vi "ReadRecords.vi"(8 "error in (no error)":errorcluster, 10 "Num records to read":i32, 11 "FpgaRef5782 in":refnum<class "FpgaRefx410.lvclass">) -> (0 "error out":errorcluster, 2 "Data":dbl[][](array[numeric]), 3 "FpgaRef5782 out":refnum<class "FpgaRefx410.lvclass">)   [LabVIEW 2025, in "FpgaRefx410.lvclass"]
uses:
  FpgaRefx410.lvclass
  FpgaRefx410.lvclass/FpgaRefx410.ctl
  <vilib>/Utility/error.llb/Error Cluster From Error Code.vi
  <vilib>/rvi/errors/niLvFpgaAdjustHostInterfaceError.vi
  <vilib>/rvi/interface/nirviMethod/nirviMethod.xnode
  x410 FPGA ref.ctl
  <vilib>/FPGAPlugInAG/Dynamic/niLvFpga_ReadFifo_Dynamic.vi
  <vilib>/rvi/errors/niLvFpgaMergeErrorWithErrorCode.vi
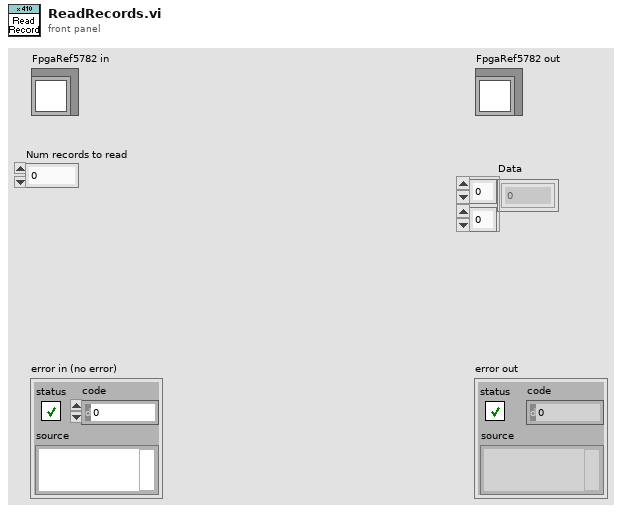
[diagram p1: front panel]
types:
  T1 = typedef "x410 FPGA ref.ctl" = refnum<k20>
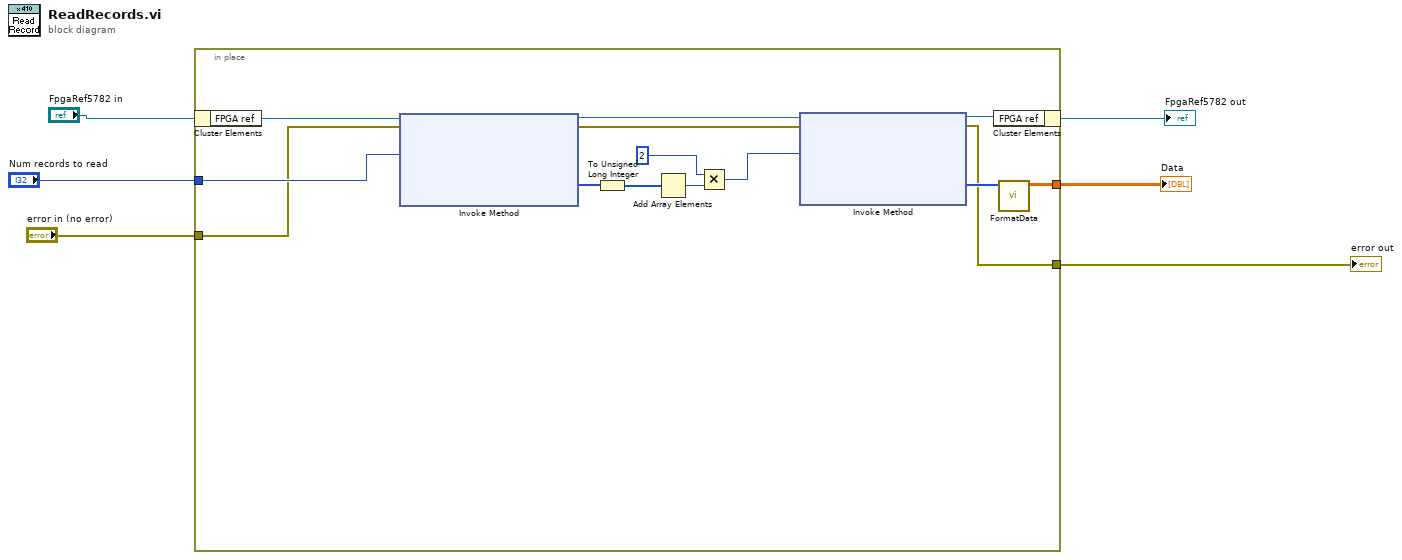
[diagram p0: block diagram]
diagram:
  n1 = in-place {
    in-place-border: "Num records to read" -> [w19]
    in-place-border: "error in (no error)" -> [w18]
    in-place-border: [w9] -> w2
    in-place-border: [w7] -> w1
    n2 = in-place-cluster #1("FpgaRef5782 in") -> ("FPGA ref"=w20:T1)
    n3 = xnode "Invoke Method"("FPGA VI Reference In"=w20, "error in"=w18, "Number of Elements"=w19) -> ("FPGA VI Reference Out"=w13:T1, "error out"=w8:errorcluster, "Data"=w17:u16[])  [unwired: 1 in, 1 out]
    n4 = To Unsigned Long Integer(number=w17) -> (unsigned 32bit integer=w16:u32[])
    n5 = Add Array Elements(numeric array=w16) -> (sum=w15:u32)
    n6 = Multiply(x=u32 2, y=w15) -> (x*y=w12:u32)
    n7 = xnode "Invoke Method"("FPGA VI Reference In"=w13, "error in"=w8, "Number of Elements"=w12) -> ("FPGA VI Reference Out"=w11:T1, "error out"=w7:errorcluster, "Data"=w10:u64[])  [unwired: 1 in, 1 out]
    n8 = in-place-cluster #1("FPGA ref"=w11) -> (→"FpgaRef5782 out":refnum<class "FpgaRefx410.lvclass">)
    n9 = call "FormatData.vi"("Raw data"=w10) -> ("Scaled"=w9:dbl[][])  [unwired: 10 in]
  }
  "error out" <- w1
  "Data" <- w2
